vi "Row Col To Range.vi"(1 "Column":i32, 2 "Row":i32) -> (0 "Output String":string)   [LabVIEW 2010, in "NI_ReportGenerationToolkit.lvlib"]
doc: "Convert Row number and Column number into Excel Format of A1, A2,.. B1, B2.... and so on."
uses:
  <vilib>/addons/_office/NI_ReportGenerationToolkit.lvlib
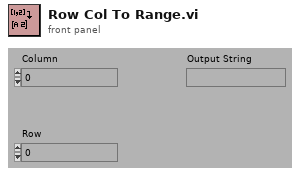
[diagram p1: front panel]
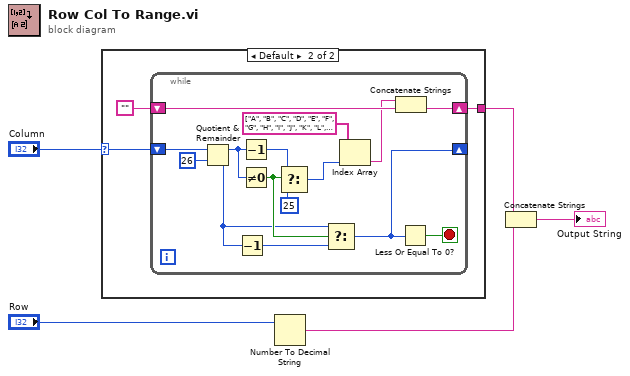
[diagram p0: block diagram]
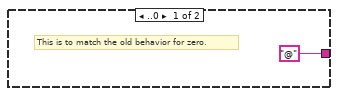
[diagram p2: hidden frame]
diagram:
  n1 = case shown="Default" "Column" {
    selector: "Column" -> [_ w7]
    tunnel: ["@" w8] -> w3
    frame ..0 {
      # "This is to match the old behavior for zero."
    }
    frame Default {
      n2 = while {
        shift-right: [w22] -> w8
        shift-left: "" -> [w19]
        shift-right: [w12] -> _
        shift-left: w7 -> [w23]
        stop <- w21 stop-if-true
        n3 = Quotient & Remainder(x=w23, y=26) -> (x-y*floor(x/y)=w15:i32, floor(x/y)=w10:i32)
        n4 = Decrement(x=w10) -> (x-1=w13:i32)
        n5 = Decrement(x=w15) -> (x-1=w17:i32)
        n6 = Not Equal To 0?(x=w15) -> (x != 0?=w14:bool)
        n7 = Select(t=w17, s=w14, f=25) -> (s? t:f=w16:i32)
        n8 = Select(t=w10, s=w14, f=w13) -> (s? t:f=w12:i32)
        n9 = Index Array(array=string[] ["A", "B", "C", "D", "E", "F", "G", "H", "I", "J", "K", "L", "M", "N", "O", "P", "Q", "R", "S", "T", "U", "V", "W", "X", "Y", "Z"], index=w16) -> (element=w18:string)
        n10 = Concatenate Strings(w18, w19) -> (w22:string)
        n11 = Less Or Equal To 0?(x=w12) -> (x <= 0?=w21:bool)
      }
    }
  }
  n12 = Number To Decimal String(number="Row") -> (decimal integer string=w4:string)  [unwired: 1 out]
  n13 = Concatenate Strings(w3, w4) -> (→"Output String":string)
